vi "Meter-TestMain.vi"() -> ()   [LabVIEW 2013, in "Meter-Test.lvclass"]
uses:
  Meter-Test.lvclass
panel:
  in  "Meter-Test.lvclass":refnum<class "Meter-Test.lvclass">
  out "Meter-Test out":refnum<class "Meter-Test.lvclass">
  out "List of Meters that Failed":string
  out "Meter Test Pass or Fail":bool
  in  "Error":errorcluster
  out "Error":errorcluster
  # "Inputs"
  # "Outputs"
  # "Create User Interface to here to let the user\nknow if the meter test passed or failed"
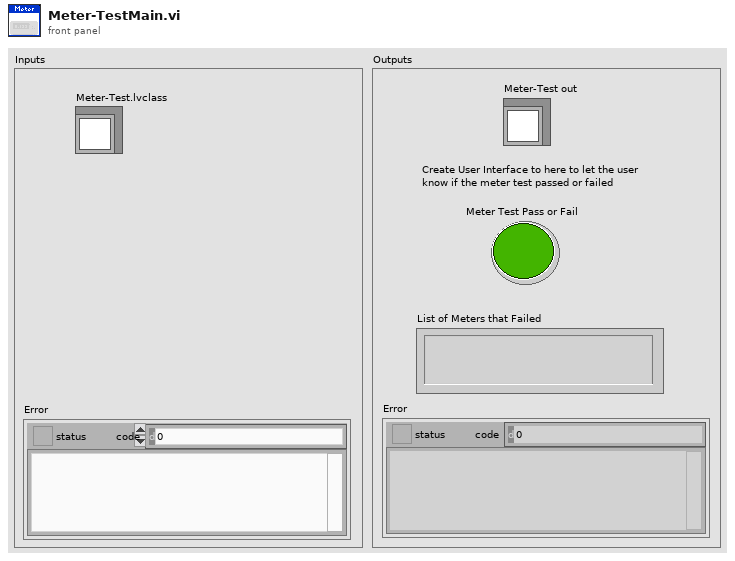
[diagram p1: front panel]
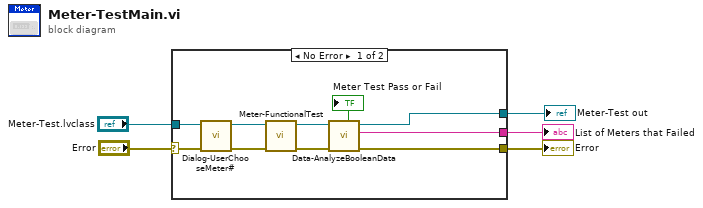
[diagram p0: block diagram]
diagram:
  n1 = case shown="No Error" "Error" {
    selector: "Error" -> [w6 w17]
    tunnel: "Meter-Test.lvclass" -> [w15 w16]
    tunnel: [w9 w17] -> w4
    tunnel: [w8 _] -> w3
    tunnel: [w7 w16] -> w2
    frame No Error {
      n2 = call "Dialog-UserChooseMeter#.vi"("error in (no error)"=w6, "Meter-Test in"=w15) -> ("error out"=w13:errorcluster, "Meter-Test out"=w14:refnum<class "Meter-Test.lvclass">)  [unwired: 8 in]
      n3 = call "Meter-FunctionalTest.vi"("error in (no error)"=w13, "Meter-Test in"=w14) -> ("error out"=w11:errorcluster, "Meter-Test out"=w12:refnum<class "Meter-Test.lvclass">)  [unwired: 8 in]
      n4 = call "Data-AnalyzeBooleanData.vi"("error in (no error)"=w11, "Meter-Test in"=w12) -> ("error out"=w9:errorcluster, "Meters That Failed"=w8:string, "Meter-Test out"=w7:refnum<class "Meter-Test.lvclass">, "Meter Test Passed or Failed"=→"Meter Test Pass or Fail":bool)  [unwired: 6 in]
    }
    frame Error {
    }
  }
  "Error" <- w4
  "List of Meters that Failed" <- w3
  "Meter-Test out" <- w2
